vi "y.vi"() -> ()   [LabVIEW 2018]
uses:
  Message.ctl
  States.ctl
  <vilib>/NI/STM/SubVIs/MetaDataElement.ctl
  <vilib>/NI/STM/TCP/TCP Read Options.ctl
  <vilib>/NI/STM/TCP/TCP Write Options.ctl
  <vilib>/NI/STM/TCP/Write Meta Data (TCP Ref).vi
  <vilib>/NI/STM/TCP/Get Connection Reference (TCP).vi
  <vilib>/NI/STM/TCP/Write Meta Data (TCP Clst).vi
  <vilib>/NI/STM/TCP/Write Message (TCP).vi
  <vilib>/NI/STM/TCP/Read Message (TCP).vi
  <vilib>/NI/STM/NI STM.lvlib
panel:
  in  "Server IP":string="192.168.43.226"
  out "Status":string="Connecting"
  out "Illuminance [lux]":dbl
  in  "Measure":bool
  in  "Stop Button":bool
  in  "Blue LED":u8(slide) scale=0.0..100.0
  in  "Green LED":u8(slide) scale=0.0..100.0
  in  "Red LED":u8(slide) scale=0.0..100.0
  in  "White LED":u8(slide) scale=0.0..100.0
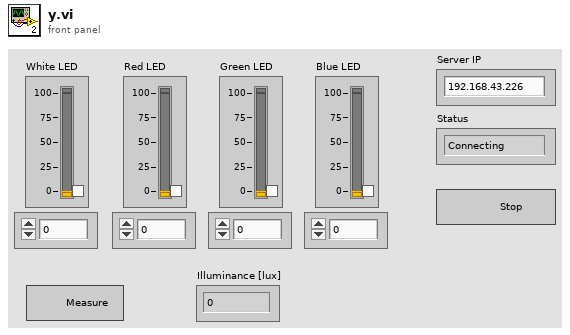
[diagram p1: front panel]
types:
  T1 = typedef "NI STM.lvlib/MetaDataElement.ctl" = string
  T2 = typedef "Message.ctl" = cluster{"States":T3, "Data":variant}
  T3 = typedef "States.ctl" = enum16{"Set LEDs", "Measure", "Exit"}
  T4 = typedef "NI STM.lvlib/TCP Connection Info.ctl" = cluster{"connection ID":refnum<k5>, "meta data":T1[]}
  T5 = typedef "NI STM.lvlib/TCP Read Options.ctl" = cluster{"ignore timeout error":bool, "timeout ms (1000)":i32}
  T6 = typedef "NI STM.lvlib/TCP Write Options.ctl" = cluster{"ignore timeout error":bool, "timeout ms (1000)":i32}
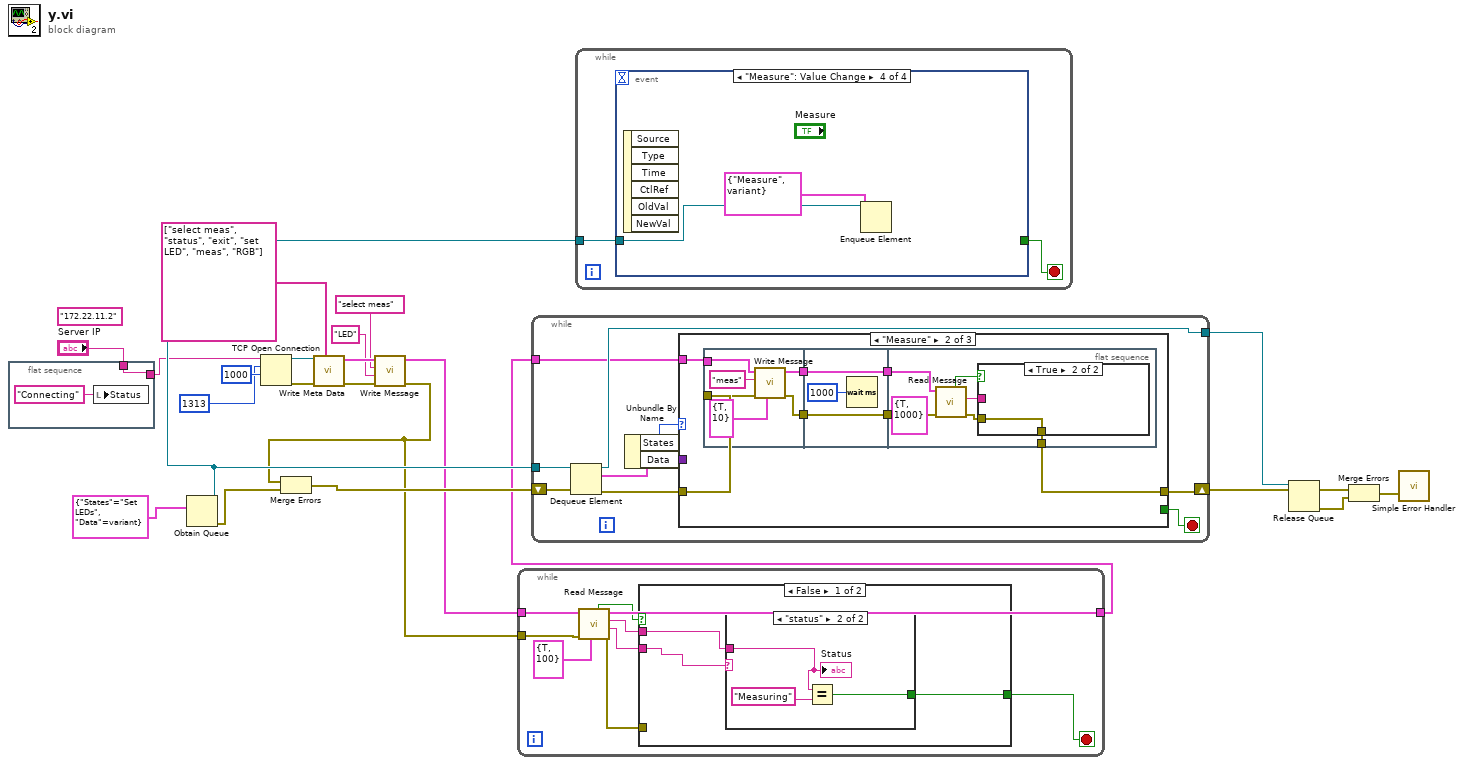
[diagram p0: block diagram]
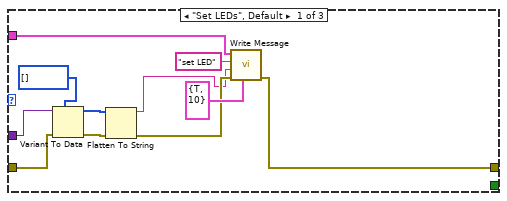
[diagram p4: hidden frame]
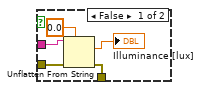
[diagram p5: hidden frame]
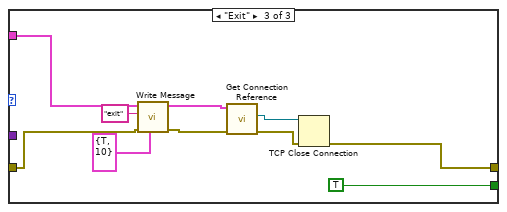
[diagram p6: hidden frame]
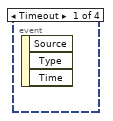
[diagram p7: hidden frame]
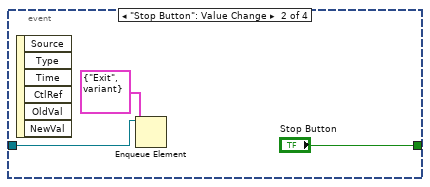
[diagram p8: hidden frame]
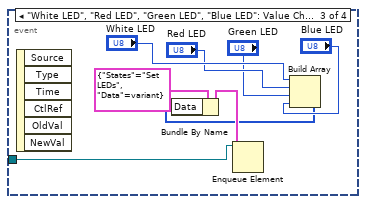
[diagram p9: hidden frame]
diagram:
  (unwired) "172.22.11.2" ("address")
  n1 = flat-sequence {
    tunnel: "Server IP" -> [w23]
    tunnel: [w23] -> w1
    frame #0 {
      n2 = local write "Status"("Connecting" ("Status")) -> ()
    }
  }
  n3 = Obtain Queue(element data type=T2 {"States"=enum."Set LEDs", "Data"=variant} ("Message")) -> (queue out=w16:refnum<queue>, error out=w17:errorcluster)  [unwired: 4 in, 1 out]
  n4 = TCP Open Connection(address=w1, remote port or service name=u16 1313, timeout ms (60000)=1000) -> (connection ID=w19:refnum<k5>, error out=w20:errorcluster)  [unwired: 2 in]
  n5 = call-poly <vilib>:"Write Meta Data.vi"("meta data"=T1[] ["select meas", "status", "exit", "set LED", "meas", "RGB"], "error in"=w20, "connection ID"=w19) -> ("error out"=w9:errorcluster, "connection info out"=w8:T4)  [unwired: 7 in]
  n6 = call-poly <vilib>:"Write Message.vi"("error in"=w9, "data"="LED", "name"="select meas", "connection info in"=w8) -> ("error out"=w3:errorcluster, "connection info out"=w5:T4)  [unwired: 6 in]
  n7 = Merge Errors(w3, w17) -> (w15:errorcluster)
  n8 = while {
    tunnel: w5 -> [w33]
    tunnel: [w32] -> w4
    tunnel: w3 -> [w30]
    stop <- w26 stop-if-true
    n9 = call-poly <vilib>:"Read Message.vi"("options"=T5 {"ignore timeout error"=TRUE, "timeout ms (1000)"=100}, "error in"=w30, "connection info in"=w33) -> ("error out"=w25:errorcluster, "name"=w27:T1, "data string"=w28:string, "connection info out"=w32:T4, "timed out?"=w29:bool)  [unwired: 3 in, 1 out]
    n10 = case shown="False" w29 {
      tunnel: w28 -> [w35 _]
      tunnel: w27 -> [w34 _]
      tunnel: [w36 _] -> w26
      tunnel: w25 -> [_ _]
      frame False {
        n11 = case shown="\"status\"" w34 {
          tunnel: w35 -> [_ w39]
          tunnel: [_ w38] -> w36
          frame Default {
          }
          frame "status" {
            n12 = Equal?(x=w39, y="Measuring") -> (x = y?=w38:bool)
            "Status" <- w39
          }
        }
      }
      frame True {
      }
    }
  }
  n13 = while {
    tunnel: w16 -> [w48]
    shift-right: [w42] -> w14
    shift-left: w15 -> [w49]
    tunnel: w4 -> [w40]
    tunnel: [w41] -> w13
    stop <- w45 stop-if-true
    n14 = Dequeue Element(queue=w48, error in (no error)=w49) -> (queue out=w41:refnum<queue>, element=w47:T2, error out=w44:errorcluster)  [unwired: 1 in, 1 out]
    n15 = Unbundle By Name(w47) -> ("States"=w46:T3, "Data"=w43:variant)
    n16 = case shown="\"Measure\"" w46 {
      tunnel: [_ _ TRUE] -> w45
      tunnel: w44 -> [w60 w66 w95]
      tunnel: w43 -> [w59 _ _]
      tunnel: [w50 w61 w96] -> w42
      tunnel: w40 -> [w55 w67 w94]
      frame "Set LEDs", Default {
        n17 = Variant To Data(error in=w60, type=u8[] [], Variant=w59) -> (data=w54:u8[], error out=w53:errorcluster)
        n18 = Flatten To String(anything=w54, error in (no error)=w53) -> (data string=w51:string, error out=w52:errorcluster)  [unwired: 2 in, 1 out]
        n19 = call-poly <vilib>:"Write Message.vi"("options"=T6 {"ignore timeout error"=TRUE, "timeout ms (1000)"=10}, "error in"=w52, "data"=w51, "name"="set LED", "connection info in"=w55) -> ("error out"=w50:errorcluster)  [unwired: 5 in, 1 out]
      }
      frame "Measure" {
        n20 = flat-sequence {
          tunnel: w67 -> [w72]
          tunnel: w66 -> [w71]
          tunnel: [w70] -> w64
          tunnel: [w69] -> w62
          tunnel: [w75] -> w65
          tunnel: w64 -> [w75]
          tunnel: [w74] -> w63
          tunnel: w62 -> [w74]
          tunnel: w65 -> [w83]
          tunnel: w63 -> [w82]
          tunnel: [w77] -> w61
          frame #0 {
            n21 = call-poly <vilib>:"Write Message.vi"("options"=T6 {"ignore timeout error"=TRUE, "timeout ms (1000)"=10}, "error in"=w71, "name"="meas", "connection info in"=w72) -> ("error out"=w69:errorcluster, "connection info out"=w70:T4)  [unwired: 6 in]
          }
          frame #1 {
            n22 = Wait (ms)(milliseconds to wait=u32 1000) -> ()  [unwired: 1 out]
          }
          frame #2 {
            n23 = call-poly <vilib>:"Read Message.vi"("options"=T5 {"ignore timeout error"=TRUE, "timeout ms (1000)"=1000}, "error in"=w82, "connection info in"=w83) -> ("error out"=w78:errorcluster, "data string"=w80:string, "timed out?"=w81:bool)  [unwired: 3 in, 3 out]
            n24 = case shown="True" w81 {
              tunnel: w80 -> [w87 _]
              tunnel: w78 -> [w88 w89]
              tunnel: [w84 w89] -> w77
              frame False {
                n25 = Unflatten From String(type=0.0, binary string=w87, error in (no error)=w88) -> (value=→"Illuminance [lux]":dbl, error out=w84:errorcluster)  [unwired: 2 in, 1 out]
              }
              frame True {
              }
            }
          }
        }
      }
      frame "Exit" {
        n26 = call-poly <vilib>:"Write Message.vi"("options"=T6 {"ignore timeout error"=TRUE, "timeout ms (1000)"=10}, "error in"=w95, "name"="exit", "connection info in"=w94) -> ("error out"=w93:errorcluster, "connection info out"=w92:T4)  [unwired: 6 in]
        n27 = call-poly <vilib>:"Get Connection Reference.vi"("error in"=w93, "connection info in"=w92) -> ("error out"=w98:errorcluster, "connection ID out"=w97:refnum<k5>)  [unwired: 7 in, 1 out]
        n28 = TCP Close Connection(connection ID=w97, error in (no error)=w98) -> (error out=w96:errorcluster)  [unwired: 1 in, 1 out]
      }
    }
  }
  n29 = while {
    tunnel: w16 -> [w100]
    stop <- w101 stop-if-true
    n30 = event shown="[3] \"Measure\": Value Change" {
      selector: _ -> [_ _ _ _]
      dyn-events: _ -> [_ _ _ _]
      timeout: _ -> [_ _ _ _]
      tunnel: [_ "Stop Button" _ _] -> w101
      tunnel: w100 -> [_ w103 w111 w113]
      event Timeout {
        n31 = event-data() -> ()  [unwired: 1 in, 3 out]
      }
      event "Stop Button": Value Change {
        n32 = event-data() -> ()  [unwired: 1 in, 6 out]
        n33 = Enqueue Element(queue=w103, element=T2 {"States"=enum."Exit", "Data"=variant}) -> ()  [unwired: 2 in, 3 out]
      }
      event "White LED", "Red LED", "Green LED", "Blue LED": Value Change {
        n34 = event-data() -> ()  [unwired: 1 in, 6 out]
        n35 = Build Array("White LED", "Red LED", "Green LED", "Blue LED") -> (w105:u8[])
        n36 = Bundle By Name(cluster=T2 {"States"=enum."Set LEDs", "Data"=variant} ("element"), "Data"=w105) -> (w110:T2)
        n37 = Enqueue Element(queue=w111, element=w110) -> ()  [unwired: 2 in, 3 out]
      }
      event "Measure": Value Change {
        n38 = event-data() -> ()  [unwired: 1 in, 6 out]
        n39 = Enqueue Element(queue=w113, element=T2 {"States"=enum."Measure", "Data"=variant}) -> ()  [unwired: 2 in, 3 out]
      }
    }
  }
  n40 = Release Queue(queue=w13) -> (error out=w11:errorcluster)  [unwired: 2 in, 2 out]
  n41 = Merge Errors(w14, w11) -> (w12:errorcluster)
  n42 = call <vilib>:"Simple Error Handler.vi"("error in (no error)"=w12) -> ()  [unwired: 4 in, 5 out]
